vi "ClearTreeNode.vi"(8 "error in":errorcluster, 10 "tag":string, 11 "tree reference":refnum<vi>) -> (0 "error out":errorcluster)   [LabVIEW 2013, in "NISE_CEF_TreeControl.lvlib"]
uses:
  NISE_CEF_TreeControl.lvlib
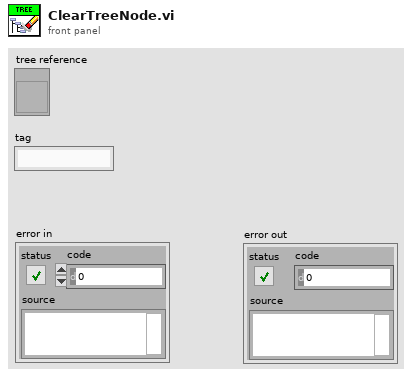
[diagram p1: front panel]
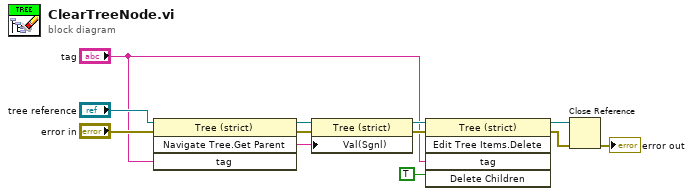
[diagram p0: block diagram]
diagram:
  n1 = invoke class="Tree (strict)" method="Navigate Tree.Get Parent"(reference="tree reference", error in="error in", "tag"="tag") -> (reference out=w8:refnum<vi>, error out=w9:errorcluster, "Navigate Tree:Get Parent"=w10:string)  [unwired: 1 in, 1 out]
  n2 = property class="Tree (strict)"(reference=w8, error in=w9, "Val(Sgnl)"=w10) -> (reference out=w12:refnum<vi>, error out=w11:errorcluster)
  n3 = invoke class="Tree (strict)" method="Edit Tree Items.Delete"(reference=w12, error in=w11, "tag"="tag", "Delete Children"=TRUE ("Delete Children?")) -> (reference out=w5:refnum<vi>, error out=w6:errorcluster)  [unwired: 1 in, 3 out]
  n4 = Close Reference(reference=w5, error in (no error)=w6) -> (error out=→"error out":errorcluster)
